vi "Run.vi"(8 "error in (no error)":errorcluster, 9 "Assembly Type":string, 10 "Control In":T1={"I-O.lvclass"=refnum, "Gantry"=refnum, "Dispenser"="COM1"}, 11 "Assembly In":refnum<class "Assembly Run.lvclass">) -> (0 "error out":errorcluster, 2 "Control Out":T1={"I-O.lvclass"=refnum, "Gantry"=refnum, "Dispenser"="COM1"}, 3 "Assembly Out":refnum<class "Assembly Run.lvclass">)   [LabVIEW 2021, in "Assembly Run.lvclass"]
uses:
  Assembly Run.lvclass
  Controller/Controllers.ctl
  Controller/I-O/I-O.lvclass
  C:/Program Files (x86)/Aerotech/A3200/LabVIEW/2010/Bin/Aerotech.A3200.dll
  Program Files (x86)/Aerotech/A3200/LabVIEW/2010/Bin/Aerotech.A3200.dll
  Assembly Run.lvclass/Assembly Run.ctl
  Workspace/Fixture.lvclass
  Routine/Routine.lvclass
  Controller/Motion/Motion.lvclass
  Controller/Controller.lvclass
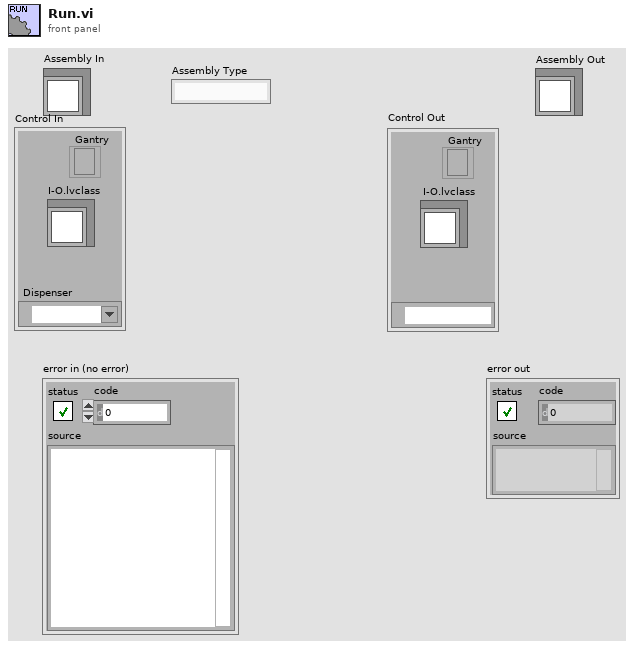
[diagram p1: front panel]
types:
  T1 = typedef "Controller.lvclass/Controllers.ctl" = cluster{"I-O.lvclass":refnum<class "I-O.lvclass">, "Gantry":refnum<k24>, "Dispenser":refnum<visa-resource-name>}
  T2 = typedef "Fixture.lvclass/Workspace.ctl" = cluster{"XYZTheta":dbl[], "Workspace Valve":i32, "Workspace Sensor":i32}
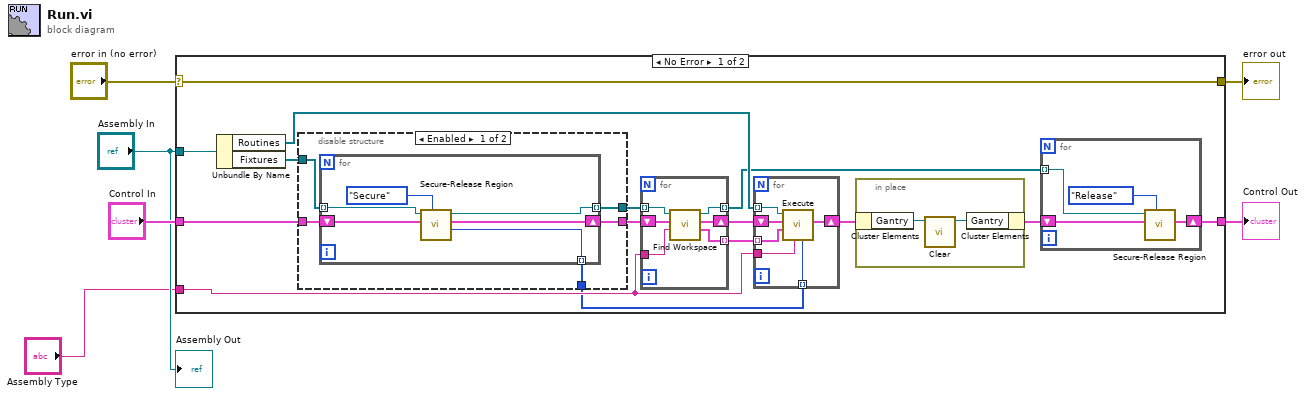
[diagram p0: block diagram]
diagram:
  n1 = case shown="No Error" "error in (no error)" {
    selector: "error in (no error)" -> [w21 w54]
    tunnel: [w21 w54] -> w5
    tunnel: [w15 w53] -> w4
    tunnel: "Assembly In" -> [w13 _]
    tunnel: "Control In" -> [w10 w53]
    tunnel: "Assembly Type" -> [w8 _]
    frame No Error {
      n2 = Unbundle By Name(w13) -> ("Routines"=w20:refnum<class "Routine.lvclass">[], "Fixtures"=w14:refnum<class "Fixture.lvclass">[])
      n3 = disable-structure shown="Enabled" {
        disable-tunnel: [w26 w34] -> w18
        disable-tunnel: w14 -> [w25 w34]
        disable-tunnel: w10 -> [w24 w33]
        disable-tunnel: [w23 w33] -> w9
        disable-tunnel: [w22 _] -> w7
        frame Enabled {
          n4 = for {
            tunnel: [w32] -> w26 mode=indexing
            tunnel: w25 -> [w31] mode=indexing
            shift-right: [w29] -> w23
            shift-left: w24 -> [w30]
            tunnel: [w27] -> w22 mode=indexing
            n5 = call-dynamic "Secure-Release Region.vi"("Action"=enum16{"Secure", "Release"}."Secure", "Control In"=w30, "Fixture in"=w31) -> ("Position"=w27:i32, "Control Out"=w29:T1, "Fixture out"=w32:refnum<class "Fixture.lvclass">)  [unwired: 5 in, 1 out]
          }
        }
        frame Disabled {
        }
      }
      n6 = for {
        tunnel: w18 -> [w52] mode=indexing
        tunnel: [w47] -> w19 mode=indexing
        tunnel: [w51] -> w17 mode=indexing
        shift-right: [w49] -> w12
        shift-left: w9 -> [w50]
        tunnel: w8 -> [w48]
        n7 = call-dynamic "Find Workspace.vi"("Assembly Type"=w48, "Control In"=w50, "Workspace In"=w52) -> (1:"Workspace Out"=w47:T2, "Control Out"=w49:T1, 3:"Workspace Out"=w51:refnum<class "Fixture.lvclass">)  [unwired: 5 in, 1 out]
      }
      n8 = for {
        tunnel: w20 -> [w46] mode=indexing
        tunnel: w19 -> [w45] mode=indexing
        shift-right: [w43] -> w11
        shift-left: w12 -> [w44]
        tunnel: w8 -> [w42]
        tunnel: w7 -> [w41] mode=indexing
        n9 = call-dynamic "Execute.vi"("Position"=w41, "Assembly Type"=w42, "Workspace"=w45, "Control In"=w44, "Routine in"=w46) -> ("Control Out"=w43:T1)  [unwired: 4 in, 2 out]
      }
      n10 = in-place {
        n11 = in-place-cluster #1(w11) -> ("Gantry"=w39:refnum<k24>)
        n12 = call "Clear.vi"("Gantry In"=w39) -> ("Gantry Out"=w40:refnum<k24>)  [unwired: 9 in, 1 out]
        n13 = in-place-cluster #1("Gantry"=w40) -> (w16:T1)
      }
      n14 = for {
        tunnel: w17 -> [w38] mode=indexing
        shift-right: [w37] -> w15
        shift-left: w16 -> [w36]
        n15 = call-dynamic "Secure-Release Region.vi"("Action"=enum16{"Secure", "Release"}."Release", "Control In"=w36, "Fixture in"=w38) -> ("Control Out"=w37:T1)  [unwired: 5 in, 3 out]
      }
    }
    frame Error {
    }
  }
  "error out" <- w5
  "Control Out" <- w4
  "Assembly Out" <- "Assembly In"
